vi "Initialize Comm Refs.vi"(7 "max queue size (100)":i32=100, 8 "error in (no error)":errorcluster, 11 "Name":string) -> (0 "error out":errorcluster, 3 "Comm.lvclass":refnum<class "VeriStand Comm.lvclass">)   [LabVIEW 2020, in "NI VeriStand Addon Network Comm.lvlib" / "VeriStand Comm.lvclass"]
uses:
  VeriStand Comm.lvclass
  VeriStand Comm.lvclass/VeriStand Comm.ctl
  <vilib>/NI/STM/NI STM.lvlib
  <vilib>/NI/AMC/AMC.lvlib
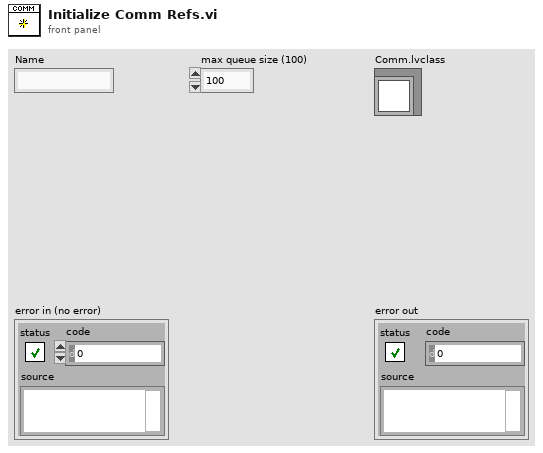
[diagram p1: front panel]
types:
  T1 = typedef "AMC.lvlib/Message Queue.ctl" = refnum<queue>
  T2 = typedef "NI STM.lvlib/TCP Connection Manager Reference.ctl" = refnum<data-value>
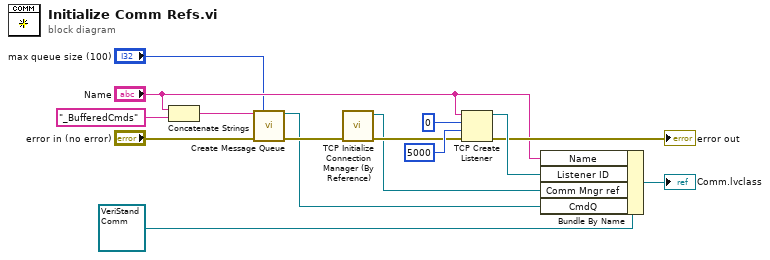
[diagram p0: block diagram]
diagram:
  n1 = Concatenate Strings("Name", "_BufferedCmds" ("string")) -> (w9:string)
  n2 = call <vilib>:"Create Message Queue.vi"("message queue name"=w9, "max queue size (-1, unlimited)"="max queue size (100)", "error in"="error in (no error)") -> ("message queue out"=w4:T1, "error out"=w5:errorcluster)  [unwired: 11 in]
  n3 = call <vilib>:"TCP Initialize Connection Manager (By Reference).vi"("error in (no error)"=w5) -> ("error out"=w12:errorcluster, "connection manager ref out"=w10:T2)  [unwired: 9 in]
  n4 = TCP Create Listener(8:w12, 9:5000 ("timeout ms (25000)"), 10:u16 0 ("port"), 11:"Name") -> (0:→"error out":errorcluster, 3:w15:refnum<k5>)  [unwired: 1 in, 1 out]
  n5 = Bundle By Name(cluster=refnum<class "VeriStand Comm.lvclass"> refnum ("NI VeriStand Addon Network Comm.lvlib:VeriStand Comm.lvclass"), "Name"="Name", "Listener ID"=w15, "Comm Mngr ref"=w10, "CmdQ"=w4) -> (→"Comm.lvclass":refnum<class "VeriStand Comm.lvclass">)
